vi "SimpleSerialTest_with_regex.vi"() -> ()   [LabVIEW 2013]
uses:
  Data/TypeDefs/Notifiers.ctl
  Data/TypeDefs/UTM Location.ctl
  Data/TypeDefs/Sail Set Suggestions.ctl
  Data/TypeDefs/Rudder Set Suggestions.ctl
  Data/TypeDefs/OverrideInformation.ctl
  Data/TypeDefs/OverrideMode.ctl
  Data/TypeDefs/MotorSetup.ctl
  Data/TypeDefs/DynamixelSetupInfo.ctl
  Data/TypeDefs/AirmarStatus.ctl
  Data/TypeDefs/HardwareOnline.ctl
  Data/TypeDefs/DynamixelCycleTracker.ctl
  Data/TypeDefs/RC Input Values.ctl
  Classes/Waypoint/Waypoint.lvclass
  <vilib>/regexp/Match Regular Expression.xnode
  <vilib>/Instr/_visa.llb/VISA Configure Serial Port (Instr).vi
  Data/TypeDefs/GPS-Compass Queue Cluster.ctl
  Data/TypeDefs/WindData Queue Cluster.ctl
panel:
  out "array":string[][](array[string])
  out "Loop Frequency":dbl(graph)
  out "Loop Frequency (Hz)":dbl
  in  "Cycles per buffer flush":i32=1000
  out "Sentence":string
  in  "stop":bool
  out "While counter":i32
  in  "NotifierReff":T1
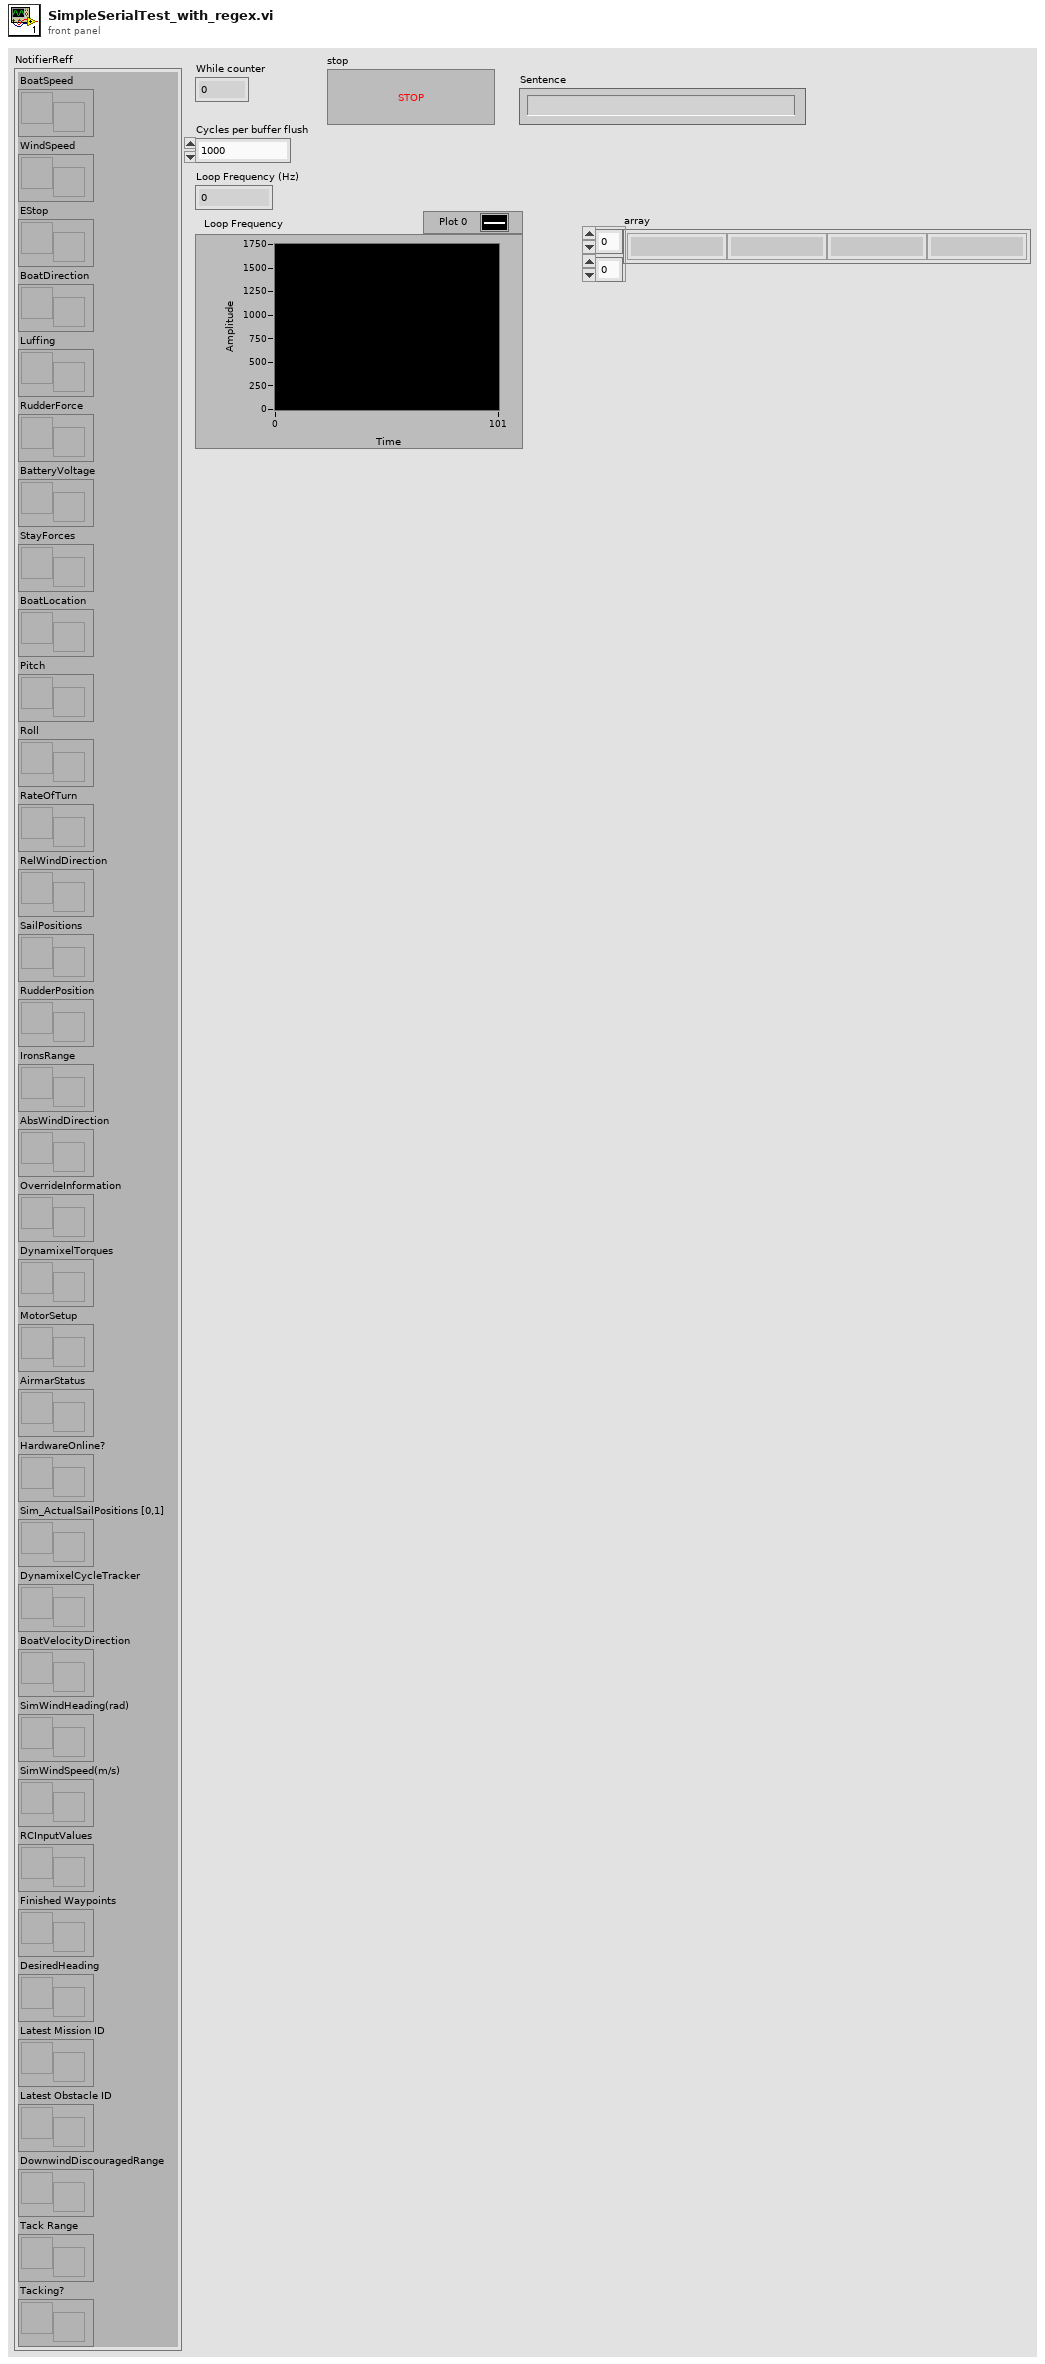
[diagram p1: front panel]
types:
  T1 = typedef "Notifiers.ctl" = cluster{"BoatSpeed":refnum<notifier>, "WindSpeed":refnum<notifier>, "EStop":refnum<notifier>, "BoatDirection":refnum<notifier>, "Luffing":refnum<notifier>, "RudderForce":refnum<notifier>, "BatteryVoltage":refnum<notifier>, "StayForces":refnum<notifier>, "BoatLocation":refnum<notifier>, "Pitch":refnum<notifier>, "Roll":refnum<notifier>, "RateOfTurn":refnum<notifier>, "RelWindDirection":refnum<notifier>, "SailPositions":refnum<notifier>, "RudderPosition":refnum<notifier>, "IronsRange":refnum<notifier>, "AbsWindDirection":refnum<notifier>, "OverrideInformation":refnum<notifier>, "DynamixelTorques":refnum<notifier>, "MotorSetup":refnum<notifier>, "AirmarStatus":refnum<notifier>, "HardwareOnline?":refnum<notifier>, "Sim_ActualSailPositions [0,1]":refnum<notifier>, "DynamixelCycleTracker":refnum<notifier>, "BoatVelocityDirection":refnum<notifier>, "SimWindHeading(rad)":refnum<notifier>, "SimWindSpeed(m/s)":refnum<notifier>, "RCInputValues":refnum<notifier>, "Finished Waypoints":refnum<notifier>, "DesiredHeading":refnum<notifier>, "Latest Mission ID":refnum<notifier>, "Latest Obstacle ID":refnum<notifier>, "DownwindDiscouragedRange":refnum<notifier>, "Tack Range":refnum<notifier>, "Tacking?":refnum<notifier>}
  T2 = typedef "WindData Queue Cluster.ctl" = cluster{"RelWindDirection Queue":refnum<queue>, "WindSpeed Queue":refnum<queue>, "AbsWindDirection Queue":refnum<queue>}
  T3 = typedef "GPS-Compass Queue Cluster.ctl" = cluster{"BoatLocation Queue":refnum<queue>, "BoatDirection Queue":refnum<queue>, "BoatSpeed Queue":refnum<queue>, "RateOfTurn Queue":refnum<queue>, "Pitch Queue":refnum<queue>, "Roll Queue":refnum<queue>, "BoatVelocityDirection Queue ":refnum<queue>}
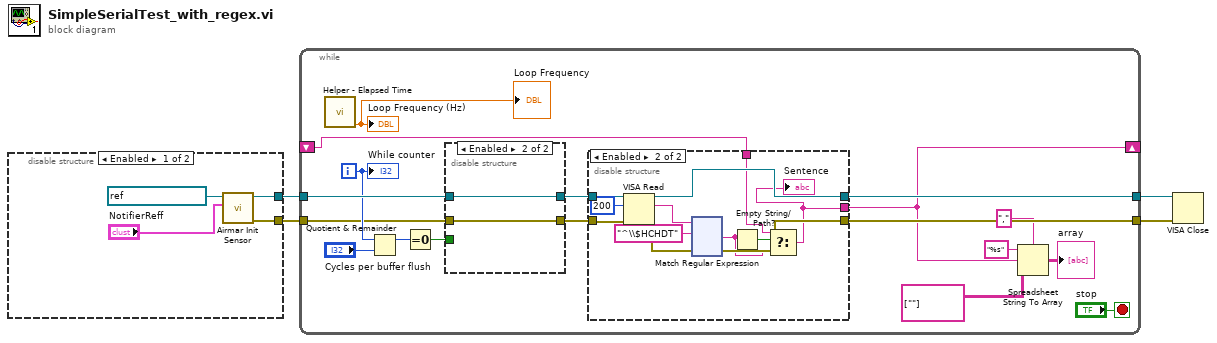
[diagram p0: block diagram]
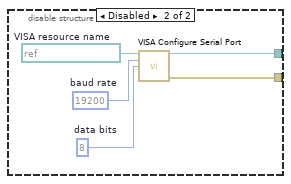
[diagram p2: hidden frame]
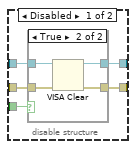
[diagram p3: hidden frame]
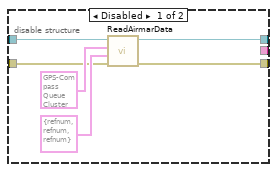
[diagram p5: hidden frame]
diagram:
  n1 = disable-structure shown="Enabled" {
    disable-tunnel: [w6 w10] -> w4
    disable-tunnel: [w5 w9] -> w2
    frame Enabled {
      n2 = call "Airmar Init Sensor.vi"("NotifierReff"="NotifierReff", "VISA Refnum in"=refnum<visa-resource-name> "ASRL2::INSTR") -> ("error out"=w5:errorcluster, "VISA Refnum out"=w6:refnum<visa-resource-name>)  [unwired: 7 in, 1 out]
    }
    frame Disabled {
      w13 = u16 8  # data bits
      w11 = u32 19200  # baud rate
      w12 = refnum<visa-resource-name> "ASRL1::INSTR"  # VISA resource name
      n3 = call-poly "VISA Configure Serial Port"("VISA resource name"=w12, "baud rate (9600)"=w11, "data bits (8)"=w13) -> ("VISA resource name out"=w10:refnum<visa-resource-name>, "error out"=w9:errorcluster)  [unwired: 11 in]
    }
  }
  n4 = while {
    tunnel: w4 -> [w30]
    tunnel: [w24] -> w3
    tunnel: w2 -> [w22]
    tunnel: [w20] -> w1
    shift-right: [w14] -> _
    shift-left: _ -> [w19]
    i -> [w29]
    stop <- "stop" stop-if-true
    n5 = call "Helper - Elapsed Time.vi"() -> ("Frequency (Hz)"=→"Loop Frequency (Hz)" →"Loop Frequency":dbl)  [unwired: 10 in, 1 out]
    n6 = Quotient & Remainder(x=w29, y="Cycles per buffer flush") -> (x-y*floor(x/y)=w28:i32)  [unwired: 1 out]
    n7 = Equal To 0?(x=w28) -> (x = 0?=w27:bool)
    n8 = disable-structure shown="Enabled" {
      disable-tunnel: [w36 w44] -> w23
      disable-tunnel: w30 -> [w35 w44]
      disable-tunnel: w27 -> [w34 _]
      disable-tunnel: w22 -> [w33 w43]
      disable-tunnel: [w32 w43] -> w21
      frame Disabled {
        n9 = case shown="True" w34 {
          tunnel: [w38 w42] -> w36
          tunnel: w35 -> [w38 w41]
          tunnel: w33 -> [w37 w40]
          tunnel: [w37 w39] -> w32
          frame False {
          }
          frame True {
            n10 = VISA Clear(VISA resource name=w41, error in (no error)=w40) -> (VISA resource name out=w42:refnum<visa-resource-name>, error out=w39:errorcluster)
          }
        }
      }
      frame Enabled {
      }
    }
    n11 = disable-structure shown="Enabled" {
      disable-tunnel: w23 -> [w50 w62]
      disable-tunnel: [w47 w57] -> w24
      disable-tunnel: w21 -> [w46 w61]
      disable-tunnel: [w45 w56] -> w20
      disable-tunnel: [_ w52] -> w14
      disable-tunnel: w19 -> [_ w51]
      frame Disabled {
        n12 = call "ReadAirmarData.vi"("Error in"=w46, "Airmar Wind Queue Cluster"=T2 {"RelWindDirection Queue"=refnum, "WindSpeed Queue"=refnum, "AbsWindDirection Queue"=refnum}, "AirmarGPS-Compass Queue Cluster"=T3 {"BoatLocation Queue"=refnum, "BoatDirection Queue"=refnum, "BoatSpeed Queue"=refnum, "RateOfTurn Queue"=refnum, "Pitch Queue"=refnum, "Roll Queue"=refnum, "BoatVelocityDirection Queue "=refnum}, "VISA UART port"=w50) -> ("Error out"=w45:errorcluster, "VISA UART port Out"=w47:refnum<visa-resource-name>)  [unwired: 5 in, 1 out]
      }
      frame Enabled {
        n13 = VISA Read(VISA resource name=w62, byte count=u32 200, error in (no error)=w61) -> (VISA resource name out=w57:refnum<visa-resource-name>, read buffer=w59:string, error out=w55:errorcluster)  [unwired: 1 out]
        n14 = xnode "Match Regular Expression"("input string"=w59, "regular expression"="^\\$HCHDT", "error in"=w55) -> ("after match"=w53:string, "error out"=w56:errorcluster)  [unwired: 3 in, 3 out]
        n15 = Empty String/Path?(string/path=w53) -> (empty?=w54:bool)
        n16 = Select(t=w51, s=w54, f=w53) -> (s? t:f=w52:string)
        "Sentence" <- w52
      }
    }
    n17 = Spreadsheet String To Array(delimiter (Tab)=",", format string="%s", spreadsheet string=w14, array type (2D Dbl)=string[][] [[""]]) -> (array=→"array":string[][])
    "While counter" <- w29
  }
  n18 = VISA Close(VISA resource name=w3, error in (no error)=w1) -> ()  [unwired: 1 out]
